vi "Kinesis - KSG101 - Get Reading.vi"() -> ()   [LabVIEW 2012]
uses:
  U:/Kinesis LabVIEW Website Examples/Thorlabs.MotionControl.Controls.dll
  Thorlabs.MotionControl.Controls.dll
  U:/Kinesis LabVIEW Website Examples/ThorLabs.MotionControl.KCube.StrainGaugeCLI.dll
  ThorLabs.MotionControl.KCube.StrainGaugeCLI.dll
panel:
  in  "Max Travel (um)":dbl
  in  "displayMode":i32(ring)=1 items=["Position"=1, "Voltage"=2, "Force"=3]
  in  "?":bool
  in  "?":bool
  out "Blocking Force":dbl
  out "Voltage":dbl
  out "Position":dbl
  in  "Serial Number":string
  in  "Max Blocking Force (N)":dbl
  in  "Max Voltage (V)":dbl
  in  "KCubeStrainGaugeControl":refnum<k24>(container)
  # "Notes:"
  # "- Ensure that the appropriate .DLLs are copied into your Project Folder. Check that the correct bit type are used depending on your version of LabVIEW\ni.e. 32-bit or 64-bit.\n\n\n\n\n\n\n\n\n\n\n\n\n\n\n- Open the example VI through the LabVIEW Project Explorer to correctly load the User Interface from Thorlabs.MotionControl.Controls.dll."
  # "Thorlabs Hardware: KSG101 - K-Cube Strain Gauge Reader\nhttps://www.thorlabs.com/thorproduct.cfm?partnumber=KSG101 \n\nDescription: This VI will enable you to connect to the KSG101 Strain Gauge Controller. This VI will call the SetDisplayMode()  which will enable you to set the current display mode to either Position, Force or Voltage mode. The GetReading() function which will return the reading between -32767 to 32768 corresponding to -100% to +100% of maximum Position, Voltage or Force. This is normalised by user specified values entered into the controls below.\n\nInstructions: \n1) Connect your KSG101 device to your PC & power the device, ensuring your stage/actutator is connected. For full device setup, the device product manual can be found on our website here. - https://www.thorlabs.com/thorproduct.cfm?partnumber=KSG101\n2) Enter the device serial number below.\n3) Enter the Max Travel, Max Voltage & Max Blocking Force of your Piezo device.\n4) Click 'Run' in the LabVIEW Toolbar.\n5) Scroll the 'displayMode' & click 'SET' to call SetDisplayMode().\n5) To close the VI, click 'END' below."
  # "Example Image of .NET Controller - VI opened via Project Explorer/ not opened via Project Explorer"
  # "VI Not Opened via Project Explorer"
  # "VI Opened via Project Explorer"
  # "- To explore the range of methods available, please visit the .NET API, included with your Kinesis software.\n\n- For tips on building your own VIs with Thorlabs Motion Control Hardware, please see our LabVIEW Guide here.\nhttps://www.thorlabs.com/newgrouppage9.cfm?objectgroup_id=10285"
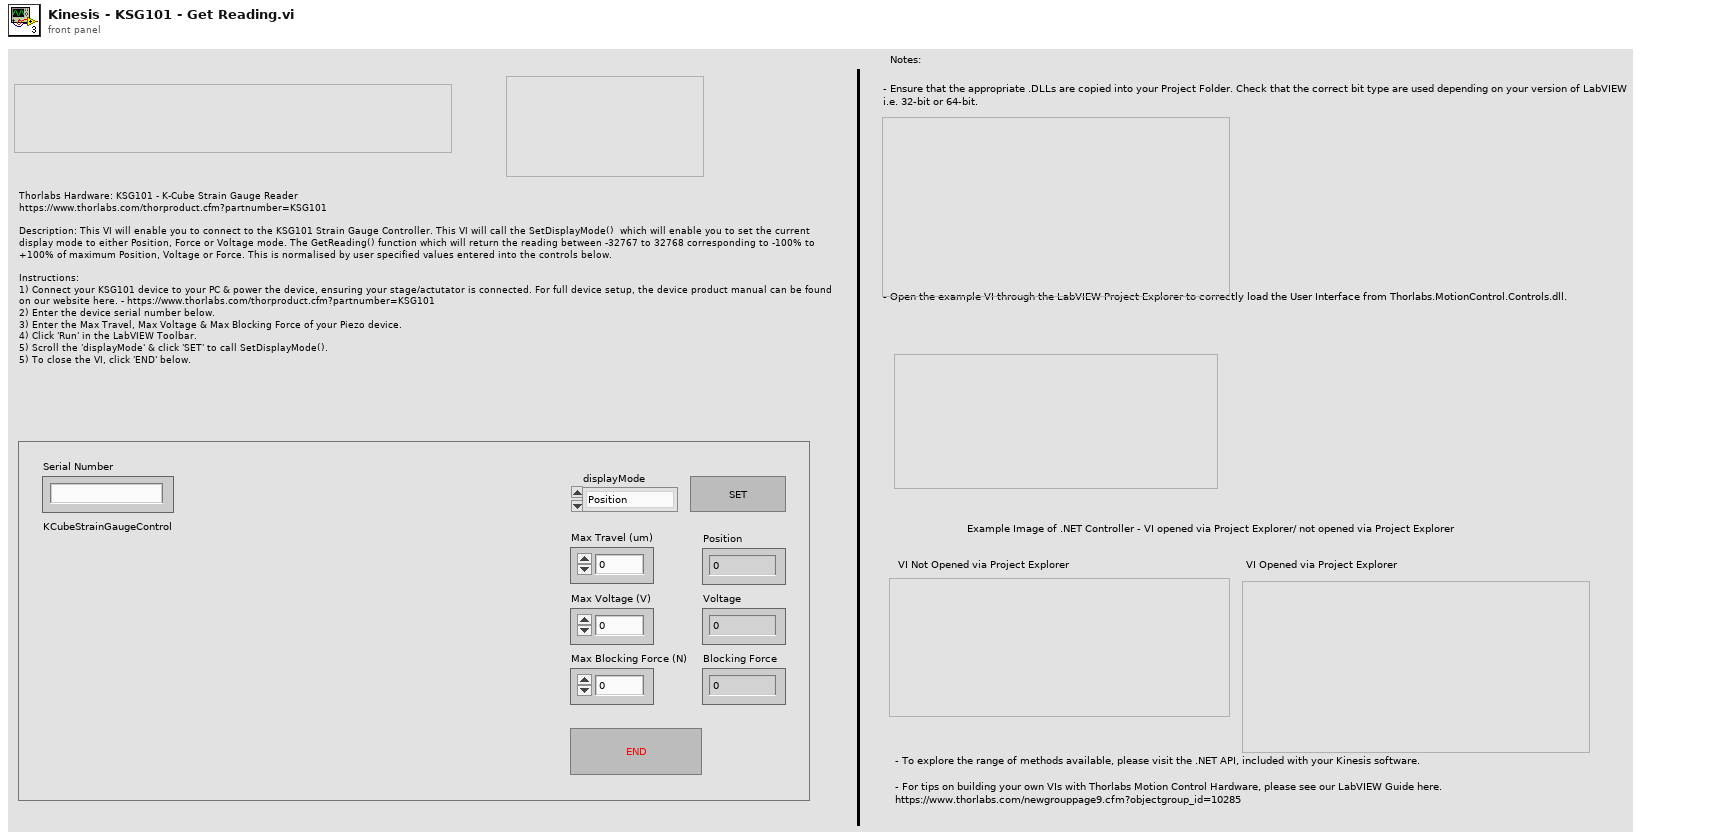
[diagram p1: front panel]
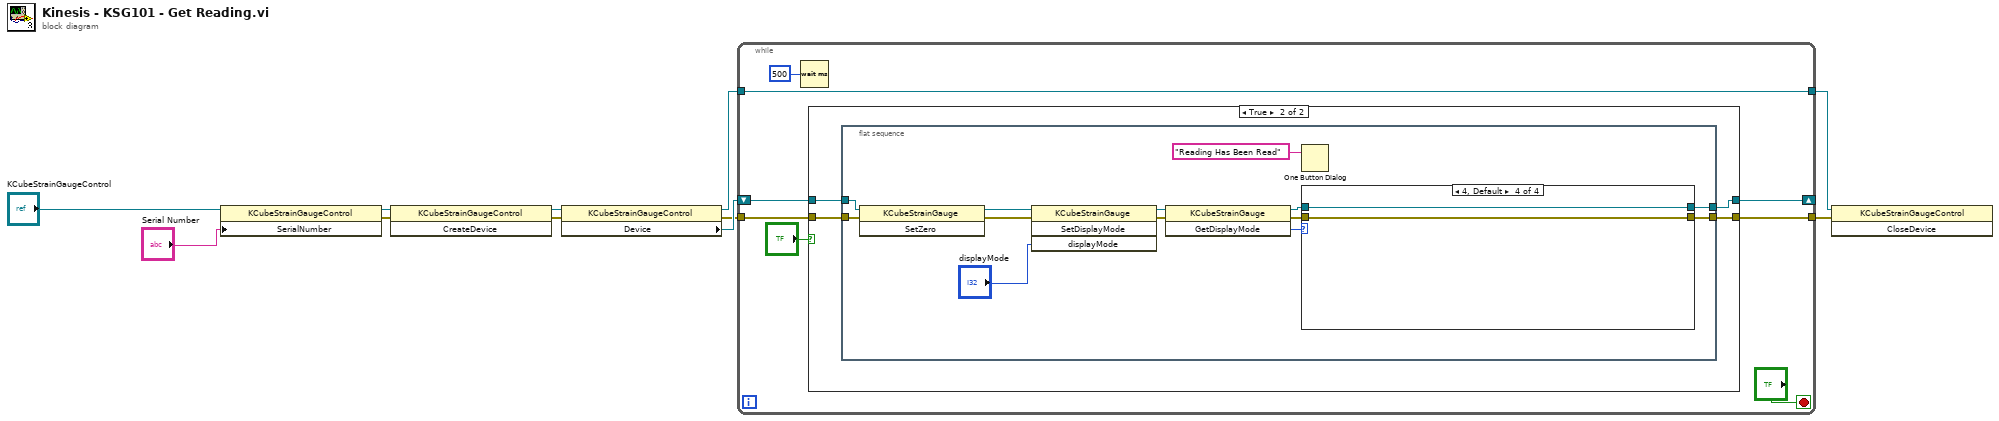
[diagram p0: block diagram]
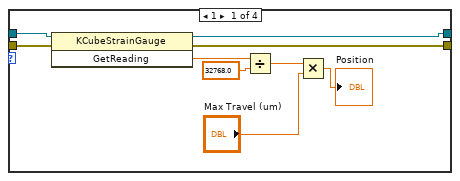
[diagram p3: hidden frame]
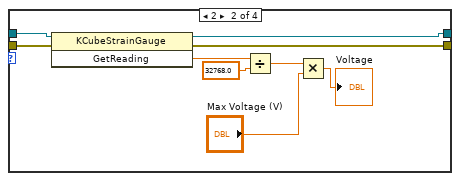
[diagram p4: hidden frame]
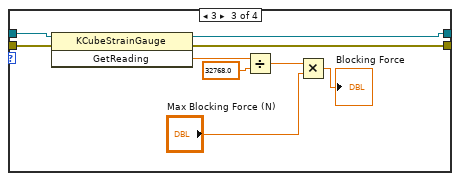
[diagram p5: hidden frame]
diagram:
  n1 = property class="KCubeStrainGaugeControl"(reference="KCubeStrainGaugeControl", "SerialNumber"="Serial Number") -> (reference out=w7:refnum<k24>, error out=w5:errorcluster)  [unwired: 1 in]
  n2 = invoke class="KCubeStrainGaugeControl" method="CreateDevice"(reference=w7, error in=w5) -> (reference out=w11:refnum<k24>, error out=w10:errorcluster)  [unwired: 1 in, 1 out]
  n3 = property class="KCubeStrainGaugeControl"(reference=w11, error in=w10) -> (reference out=w2:refnum<k24>, error out=w4:errorcluster, "Device"=w9:refnum<k24>)
  n4 = while {
    shift-right: [w18] -> _
    shift-left: w9 -> [w19]
    tunnel: w4 -> [w14]
    tunnel: [w13] -> w3
    tunnel: w2 -> [w13]
    tunnel: [w12] -> w1
    stop <- "?" stop-if-true
    n5 = Wait (ms)(milliseconds to wait=u32 500) -> ()  [unwired: 1 out]
    n6 = case shown="True" "?" {
      tunnel: w14 -> [w21 w25]
      tunnel: [w21 w24] -> w12
      tunnel: w19 -> [w20 w23]
      tunnel: [w20 w22] -> w18
      frame False {
      }
      frame True {
        n7 = flat-sequence {
          tunnel: w25 -> [w38]
          tunnel: [w36] -> w24
          tunnel: w23 -> [w35]
          tunnel: [w29] -> w22
          frame #0 {
            n8 = invoke class="KCubeStrainGauge" method="SetZero"(reference=w35, error in=w38) -> (reference out=w34:refnum<k24>, error out=w37:errorcluster)  [unwired: 1 in, 1 out]
            n9 = invoke class="KCubeStrainGauge" method="SetDisplayMode"(reference=w34, error in=w37, "displayMode"="displayMode") -> (reference out=w33:refnum<k24>, error out=w31:errorcluster)  [unwired: 1 in, 2 out]
            n10 = invoke class="KCubeStrainGauge" method="GetDisplayMode"(reference=w33, error in=w31) -> (reference out=w32:refnum<k24>, error out=w30:errorcluster, "GetDisplayMode"=w27:i32)  [unwired: 1 in]
            n11 = One Button Dialog(message="Reading Has Been Read") -> ()  [unwired: 1 in, 1 out]
            n12 = case shown="4, Default" w27 {
              tunnel: w30 -> [w46 w56 w64 w66]
              tunnel: [w45 w55 w63 w66] -> w36
              tunnel: w32 -> [w47 w54 w65 w67]
              tunnel: [w43 w50 w59 w67] -> w29
              frame 1 {
                n13 = invoke class="KCubeStrainGauge" method="GetReading"(reference=w47, error in=w46) -> (reference out=w43:refnum<k24>, error out=w45:errorcluster, "GetReading"=w42:dbl)  [unwired: 1 in]
                n14 = Divide(x=w42, y=32768.0) -> (x/y=w40:dbl)
                n15 = Multiply(x=w40, y="Max Travel (um)") -> (x*y=→"Position":dbl)
              }
              frame 2 {
                n16 = invoke class="KCubeStrainGauge" method="GetReading"(reference=w54, error in=w56) -> (reference out=w50:refnum<k24>, error out=w55:errorcluster, "GetReading"=w48:dbl)  [unwired: 1 in]
                n17 = Divide(x=w48, y=32768.0) -> (x/y=w51:dbl)
                n18 = Multiply(x=w51, y="Max Voltage (V)") -> (x*y=→"Voltage":dbl)
              }
              frame 3 {
                n19 = invoke class="KCubeStrainGauge" method="GetReading"(reference=w65, error in=w64) -> (reference out=w59:refnum<k24>, error out=w63:errorcluster, "GetReading"=w57:dbl)  [unwired: 1 in]
                n20 = Divide(x=w57, y=32768.0) -> (x/y=w61:dbl)
                n21 = Multiply(x=w61, y="Max Blocking Force (N)") -> (x*y=→"Blocking Force":dbl)
              }
              frame 4, Default {
              }
            }
          }
        }
      }
    }
  }
  n22 = invoke class="KCubeStrainGaugeControl" method="CloseDevice"(reference=w3, error in=w1) -> ()  [unwired: 1 in, 3 out]
